vi "GetMaxCounts.vi"(0 "New Image":T1) -> (1 "Maximal Value":sgl, 2 "Color":u32)   [LabVIEW 2013]
uses:
  <vilib>/vision/Image Controls.llb/IMAQ Image.ctl
  <vilib>/vision/NI_Vision_Development_Module.lvlib
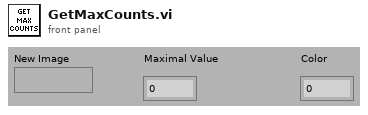
[diagram p1: front panel]
types:
  T1 = typedef "IMAQ Image.ctl" = refnum<image>
  T2 = cluster{"histogram":u32[], "Minimal Value":sgl, "Maximal Value":sgl, "Starting Value":sgl, "Interval Width":sgl, "Mean Value":sgl, "Standard  Variation":sgl, "Area (pixels)":i32}
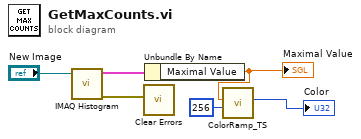
[diagram p0: block diagram]
diagram:
  n1 = call "IMAQ Histogram"("Image"="New Image") -> ("error out"=w6:errorcluster, "Histogram Report"=w2:T2)  [unwired: 9 in]
  n2 = call <vilib>:"Clear Errors.vi"("error in (no error)"=w6) -> ()  [unwired: 6 in, 1 out]
  n3 = Unbundle By Name(w2) -> ("Maximal Value"=w3:sgl)
  "Maximal Value" <- w3
  n4 = call "ColorRamp_TS.vi"("max value"=256, "value"=w3) -> ("Color"=→"Color":u32)  [unwired: 9 in]
